vi "test negative timestamp to epoch.vi"(8 "error in (no error)":errorcluster, 11 "TestCase in":refnum<class "Timestamp Tests.lvclass">) -> (0 "error out":errorcluster, 3 "TestCase out":refnum<class "Timestamp Tests.lvclass">)   [LabVIEW 2020, in "Timestamp Tests.lvclass"]
uses:
  Timestamp Tests.lvclass
  <vilib>/Utility/file.llb/Application Directory.vi
  <vilib>/Utility/libraryn.llb/Check if File or Folder Exists.vi
  <vilib>/addons/_JKI Toolkits/VI Tester/TestCase.llb/TestCase.lvclass
  C:/Program Files (x86)/National Instruments/LabVIEW 2020/vi.lib/addons/_JKI Toolkits/VI Tester/TestCase.llb/TestCase.lvclass
panel:
  out "return type":dbl format="%#_23g"
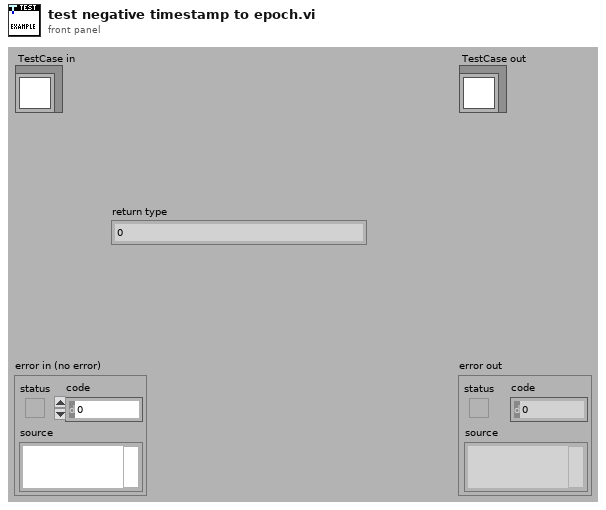
[diagram p1: front panel]
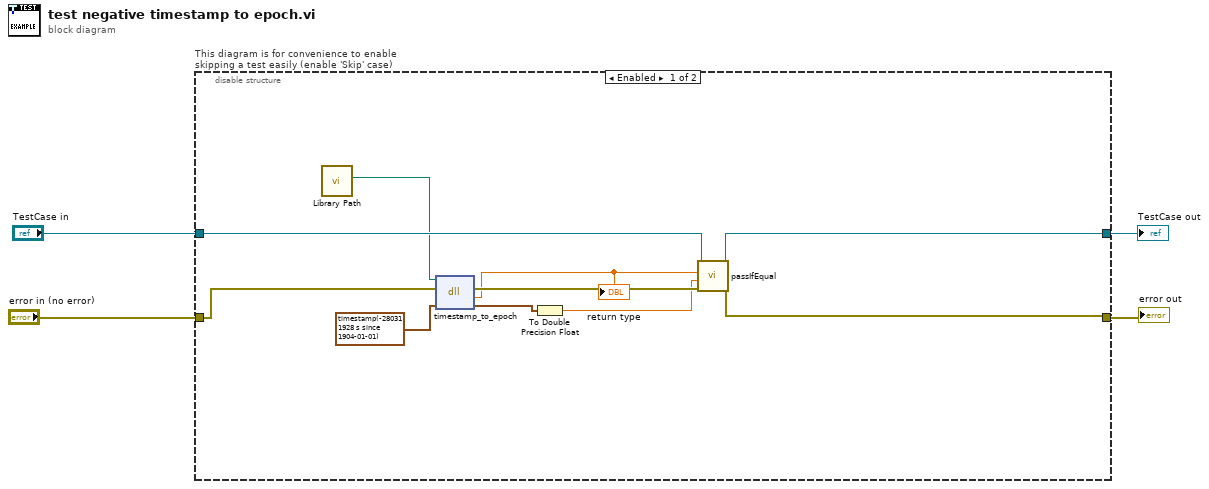
[diagram p0: block diagram]
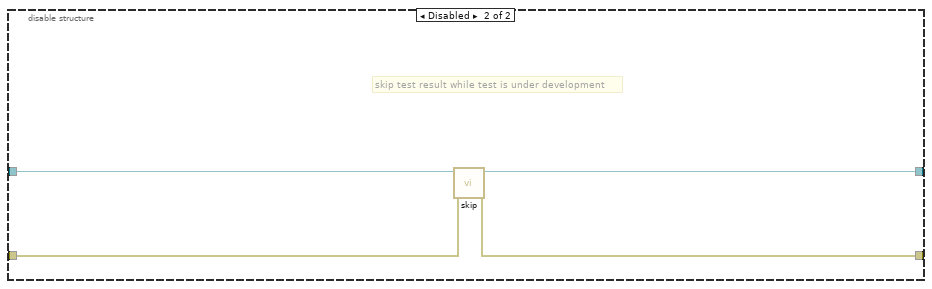
[diagram p2: hidden frame]
diagram:
  n1 = disable-structure "This diagram is for convenience to enable skipping a test easily (enable 'Skip' case)" shown="Enabled" {
    disable-tunnel: "TestCase in" -> [w14 w18]
    disable-tunnel: [w13 w16] -> w1
    disable-tunnel: [w12 w17] -> w3
    disable-tunnel: "error in (no error)" -> [w11 w15]
    frame Enabled {
      n2 = call "Library Path.vi"() -> ("Library Path"=w5:path)  [unwired: 11 in]
      n3 = dll-call lib="C:/Users/JamesMcNally/Documents/RustInterop/Rust-LabVIEW-Interop/target/debug/labview_test_library.dll" fn="timestamp_to_epoch"(path in=w5, error in=w11, "timestamp"=timestamp(-280311927.976 s since 1904-01-01) ("Time Stamp")) -> (error out=w10:errorcluster, "return type"=w6:dbl, "timestamp"=w8:timestamp)  [unwired: 1 in, 1 out]
      "return type" <- w6
      n4 = To Double Precision Float(number=w8) -> (double precision float=w7:dbl)
      n5 = call-dynamic "passIfEqual.vi"("error in (no error)"=w10, "y"=w7, "x"=w6, "TestCase in"=w14) -> ("error out"=w12:errorcluster, "TestCase out"=w13:refnum<class "Timestamp Tests.lvclass">)  [unwired: 6 in]
    }
    frame Disabled {
      # "skip test result while test is under development"
      n6 = call <vilib>:"skip.vi"("error in (no error)"=w15, "TestCase in"=w18) -> ("error out"=w17:errorcluster, "TestCase out"=w16:refnum<class "Timestamp Tests.lvclass">)  [unwired: 8 in]
    }
  }
  "error out" <- w3
  "TestCase out" <- w1
